vi "Set_Parameter_Instrument (Json).vi"(8 "error in (no error)":errorcluster caption="entrée d'erreur (pas d'erreur)", 10 "Parameter (Json)":string, 11 "Show_Result_Relay en entrée":refnum<class "Show_Result_Relay.lvclass">) -> (0 "error out":errorcluster caption="sortie d'erreur", 3 "Show_Result_Relay en sortie":refnum<class "Show_Result_Relay.lvclass">)   [LabVIEW 2020, in "Library Test.lvlib" / "Show_Result_Relay.lvclass"]
uses:
  Show_Result_Relay.lvclass
  C:/Users/ngarcin/OneDrive - Altyor/Standard TB/Class/Test/Test (Default)/Test (Default).lvclass
  Show_Result_Relay.lvclass/Show_Result_Relay.ctl
  JSON API/JSON Value/Set from JSON string.vi
  Test_Wtih_Instr/Test_With_Inst.lvclass
  JSON API/JSON Value/JSON Value.lvclass
  JSON API/Variant JSON/Variant JSON.lvlib
  JSON API/Get Polymorphic/JSON GetSet.lvlib
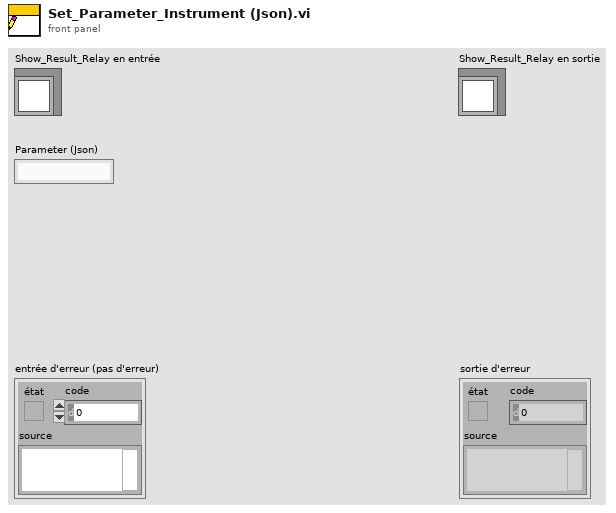
[diagram p1: front panel]
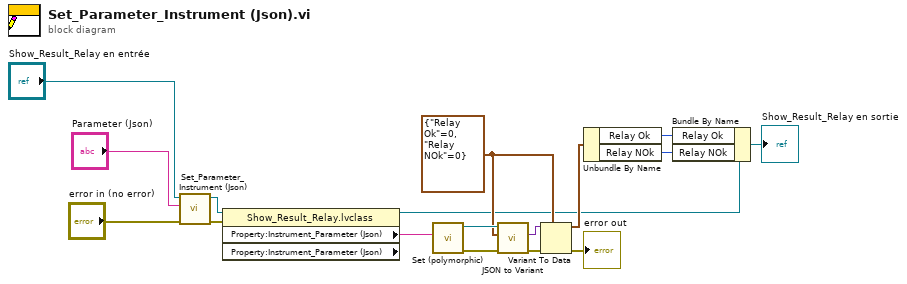
[diagram p0: block diagram]
diagram:
  w10 = cluster{"Relay Ok":u16, "Relay NOk":u16} {"Relay Ok"=0, "Relay NOk"=0} ("Cluster des données privées de classe")
  n1 = call-parent "Set_Parameter_Instrument (Json).vi"("error in (no error)"="error in (no error)", "Parameter (Json)"="Parameter (Json)", "Test (Default) en entrée"="Show_Result_Relay en entrée") -> ("error out"=w3:errorcluster, "Test (Default) en sortie"=w4:refnum<class "Show_Result_Relay.lvclass">)  [unwired: 7 in]
  n2 = property class="Show_Result_Relay.lvclass" props=["Property:Instrument_Parameter (Json)", "Property:Instrument_Parameter (Json)"](reference=w4, error in=w3) -> (reference out=w7:refnum<class "Show_Result_Relay.lvclass">, "Property:Instrument_Parameter (Json)"=w9:string)  [unwired: 2 out]
  n3 = call-poly "Set (polymorphic).vi"("JSON stream"=w9) -> ("error out"=w13:errorcluster, "JSON Value out"=w11:refnum<class "JSON Value.lvclass">)  [unwired: 8 in, 1 out]
  n4 = call "JSON to Variant.vi"("error in (no error)"=w13, "Variant (Data Type)"=w10, "JSON Value"=w11) -> ("error out"=w12:errorcluster, "Variant out"=w14:variant)  [unwired: 7 in]
  n5 = Variant To Data(error in=w12, type=w10, Variant=w14) -> (data=w8:cluster{"Relay Ok":u16, "Relay NOk":u16}, error out=→"error out":errorcluster)
  n6 = Unbundle By Name(w8) -> ("Relay Ok"=w6:u16, "Relay NOk"=w5:u16)
  n7 = Bundle By Name(cluster=w7, "Relay Ok"=w6, "Relay NOk"=w5) -> (→"Show_Result_Relay en sortie":refnum<class "Show_Result_Relay.lvclass">)
